vi "Write Handle.vi"(8 "error in":errorcluster, 10 "Session Handle":T1, 11 "Configurable Device in":refnum<class "Configurable Device.lvclass">) -> (0 "error out":errorcluster, 3 "Configurable Device out":refnum<class "Configurable Device.lvclass">)   [LabVIEW 2019, in "Configurable Device.lvclass"]
uses:
  Configurable Device.lvclass
  Reusable/Session APIs/File Access/Config Data/Config Session.ctl
  Reusable/Session APIs/File Access/Config Data/Config Data.lvclass
  Configurable Device.lvclass/Configurable Device.ctl
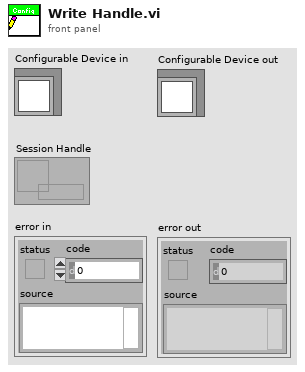
[diagram p1: front panel]
types:
  T1 = typedef "Config Data.lvclass/Config Session.ctl" = refnum<data-value>
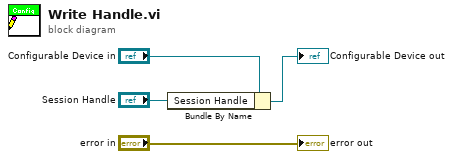
[diagram p0: block diagram]
diagram:
  n1 = Bundle By Name(cluster="Configurable Device in", "Session Handle"="Session Handle") -> (→"Configurable Device out":refnum<class "Configurable Device.lvclass">)
  "error out" <- "error in"
